vi "RefMem PtByPt Main Page.vi"(8 "error in (no error)":errorcluster, 11 "Node Ptr":T1 format="%.0x") -> (0 "error out":errorcluster)   [LabVIEW 2010, in "RefMem PtByPt Custom Device.lvlib"]
uses:
  RefMem PtByPt Custom Device.lvlib
  <vilib>/NI Veristand/Custom Device API/Custom Device Item Ref.ctl
  <vilib>/NI Veristand/Custom Device API/Path Specification.ctl
  <vilib>/NI Veristand/Custom Device API/Path Type.ctl
  <vilib>/NI Veristand/Custom Device API/Custom Device Execution Mode.ctl
  Controls/Data Channel Type.ctl
  <vilib>/NI Veristand/Custom Device API/Custom Device Channel.ctl
  <vilib>/NI Veristand/Custom Device API/Custom Device Channel Type.ctl
  Controls/Global.vi
  <vilib>/NI Veristand/Custom Device API/Get Item Property (String).vi
  <vilib>/NI Veristand/Custom Device API/Get Item Property (I32).vi
  <vilib>/NI Veristand/Custom Device API/Set Item Property (String).vi
  <vilib>/NI Veristand/Custom Device API/Set Item Property (U16).vi
  <vilib>/NI Veristand/Custom Device API/Set Item Property (I32).vi
  <vilib>/NI Veristand/Custom Device API/Custom Device API.lvlib
panel:
  in  "CPU Assignment":i32
  in  "Import":bool
  in  "Decimation":i32=1 min=1
  in  "VISA Name":string
  in  "Add Data Channel":bool
  in  "Add Data Folder":bool
  in  "Header":cluster{"Section Name":string}={"Section Name"="Reflective Memory Settings"}
  in  "Description":string
  in  "Name":string
  # "(-2 is Automatic)"
  # "(Only used if decimation >1)"
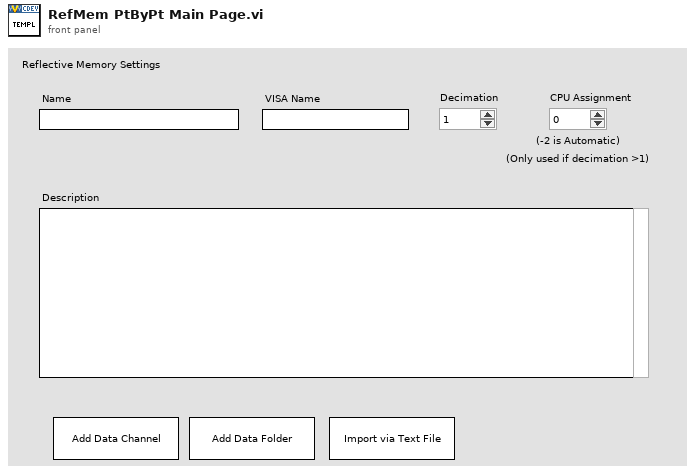
[diagram p1: front panel]
types:
  T1 = typedef "Custom Device API.lvlib/Custom Device Item Ref.ctl" = u64
  T2 = typedef "Custom Device API.lvlib/Custom Device Item Info.ctl" = cluster{"Name":string, "Is Channel":bool, "GUID":string}
  T3 = typedef "Custom Device API.lvlib/Path Specification.ctl" = cluster{"Path":path, "Type":T4}
  T4 = typedef "Custom Device API.lvlib/Path Type.ctl" = enum16{"Absolute", "To Base", "To Common Data Dir", "To Application Data Dir"}
  T5 = typedef "Custom Device API.lvlib/Custom Device Execution Mode.ctl" = enum16{"Asynchronous", "Inline HW Interface", "Inline Model Interface", "Inline Timing and Sync", "Asynchronous Timing and Sync"}
  T6 = typedef "RefMem PtByPt Custom Device.lvlib/Data Channel Type.ctl" = enum16{"Read", "Write"}
  T7 = typedef "Custom Device API.lvlib/Custom Device Channel.ctl" = cluster{"Type":T8, "Units":string, "Default Value":dbl, "Faultable":bool, "Scalable":bool}
  T8 = typedef "Custom Device API.lvlib/Custom Device Channel Type.ctl" = enum16{"Input", "Output"}
  T9 = typedef "Custom Device API.lvlib/Custom Device Commands.ctl" = enum16{"Default", "Item renamed", "Shutdown", "Dynamic button pressed"}
  T10 = typedef "Custom Device API.lvlib/Custom Device Pointer.ctl" = refnum<k24>
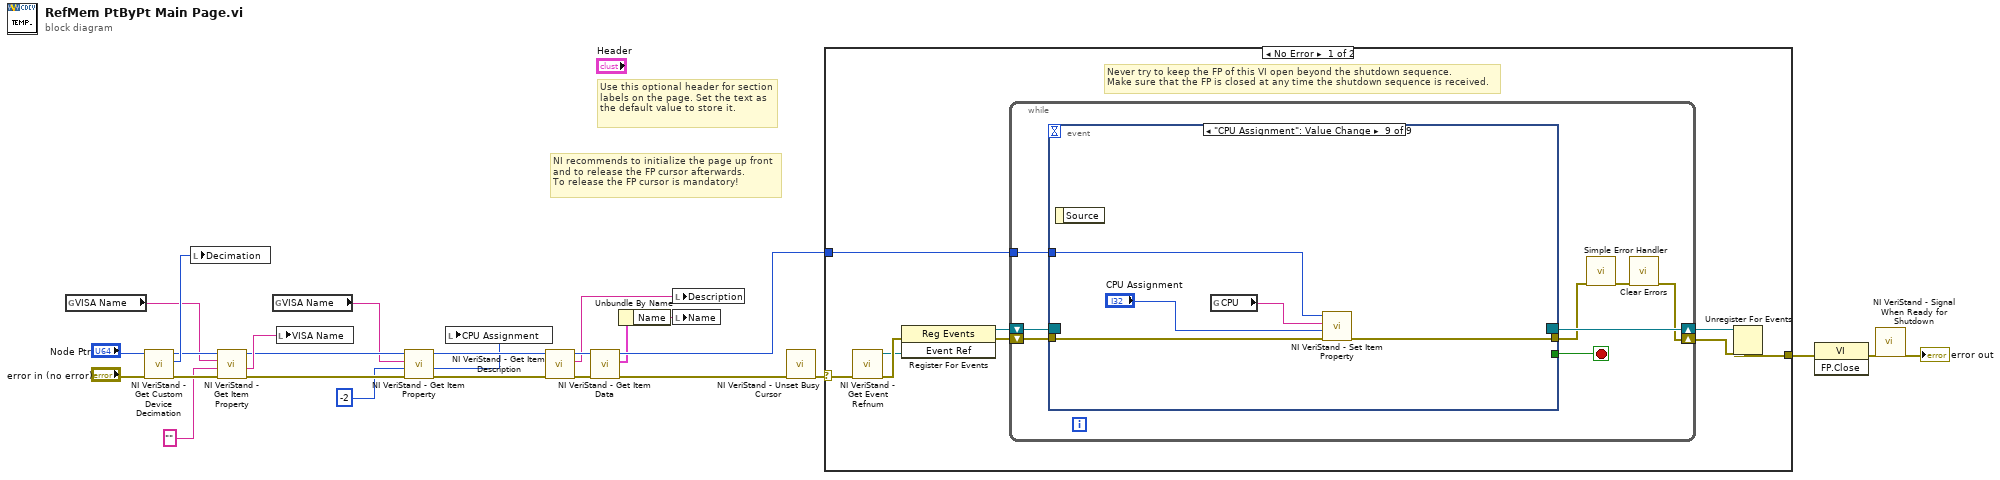
[diagram p0: block diagram]
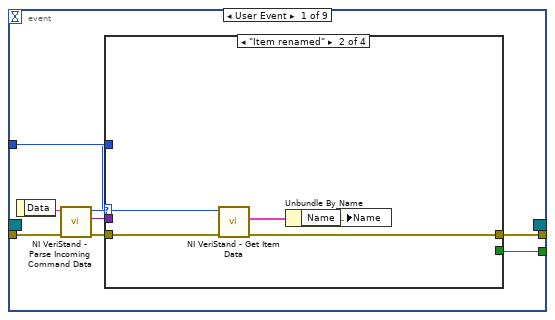
[diagram p2: hidden frame]
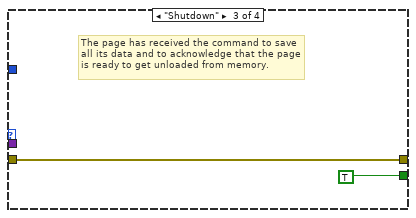
[diagram p4: hidden frame]
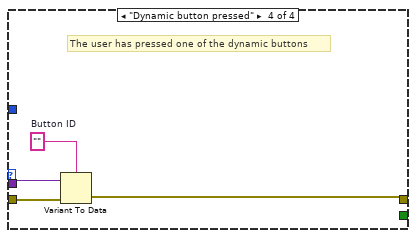
[diagram p5: hidden frame]
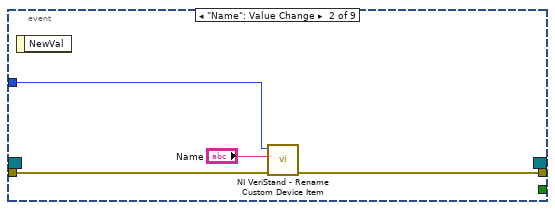
[diagram p6: hidden frame]
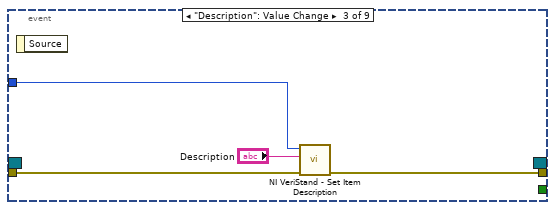
[diagram p7: hidden frame]
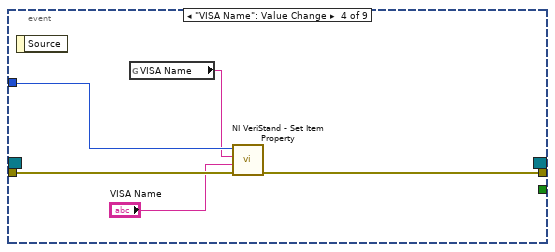
[diagram p8: hidden frame]
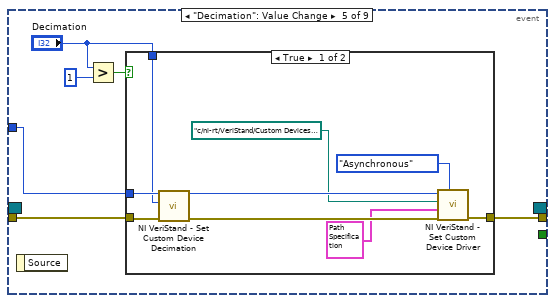
[diagram p9: hidden frame]
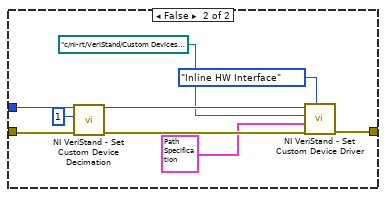
[diagram p10: hidden frame]
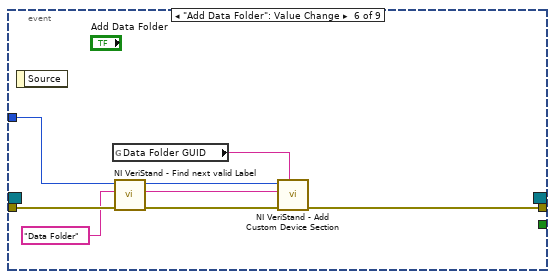
[diagram p11: hidden frame]
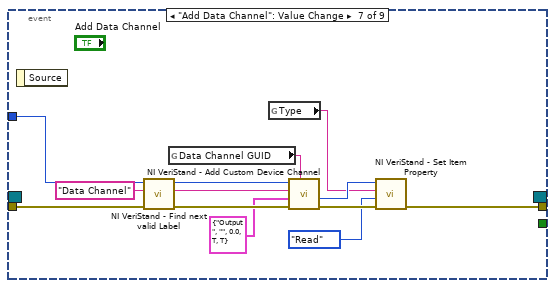
[diagram p12: hidden frame]
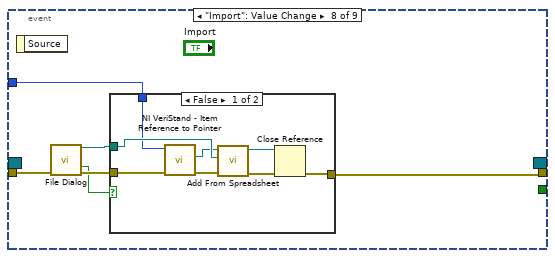
[diagram p13: hidden frame]
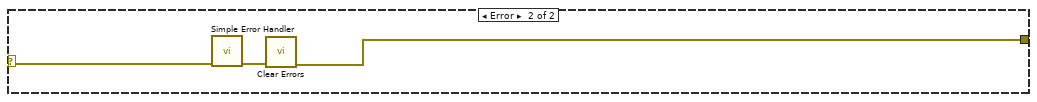
[diagram p15: hidden frame]
diagram:
  # "Use this optional header for section labels on the page. Set the text as the default value to store it."
  # "NI recommends to initialize the page up front\nand to release the FP cursor afterwards.\nTo release the FP cursor is mandatory!"
  n1 = global read "Global.vi" "VISA Name"() -> (w10:string)
  n2 = call <vilib>:"NI VeriStand - Get Custom Device Decimation.vi"("error in (no error)"="error in (no error)", "Device Ref in"="Node Ptr") -> ("error out"=w12:errorcluster, "Decimation"=w13:i32, "Device Ref out"=w11:T1)  [unwired: 7 in]
  n3 = local write "Decimation"(w13) -> ()
  n4 = call-poly <vilib>:"NI VeriStand - Get Item Property.vi"("error in (no error)"=w12, "Default Value"="" ("Section Name"), "Property Name"=w10, "Item Ref in"=w11) -> ("error out"=w7:errorcluster, "Value"=w8:string, "Item Ref out"=w6:T1)  [unwired: 4 in, 1 out]
  n5 = global read "Global.vi" "VISA Name"() -> (w5:string)
  n6 = local write "VISA Name"(w8) -> ()
  n7 = call-poly <vilib>:"NI VeriStand - Get Item Property.vi"("error in (no error)"=w7, "Default Value"=-2 ("CPU Assignment"), "Property Name"=w5, "Item Ref in"=w6) -> ("error out"=w3:errorcluster, "Value"=w1:i32, "Item Ref out"=w2:T1)  [unwired: 4 in, 1 out]
  n8 = local write "CPU Assignment"(w1) -> ()
  n9 = call <vilib>:"NI VeriStand - Get Item Description.vi"("error in (no error)"=w3, "Item Ref in"=w2) -> ("error out"=w18:errorcluster, "Description"=w19:string, "Item Ref out"=w20:T1)  [unwired: 7 out]
  n10 = call <vilib>:"NI VeriStand - Get Item Data.vi"("error in (no error)"=w18, "Item Ref in"=w20) -> ("error out"=w23:errorcluster, "Item Info"=w17:T2, "Item Ref out"=w21:T1)  [unwired: 7 out]
  n11 = Unbundle By Name(w17) -> ("Name"=w16:string)
  n12 = local write "Description"(w19) -> ()
  n13 = local write "Name"(w16) -> ()
  n14 = call <vilib>:"NI VeriStand - Unset Busy Cursor.vi"("error in (no error)"=w23) -> ("error out"=w22:errorcluster)  [unwired: 10 out]
  n15 = case shown="No Error" w22 {
    selector: w22 -> [w27 w144]
    tunnel: [w32 w142] -> w26
    tunnel: w21 -> [w28 _]
    frame No Error {
      # "Never try to keep the FP of this VI open beyond the shutdown sequence.\nMake sure that the FP is closed at any time the shutdown sequence is received."
      n16 = call <vilib>:"NI VeriStand - Get Event Refnum.vi"("error in (no error)"=w27) -> ("error out"=w35:errorcluster, "Event Ref"=w31:refnum<user-event>)  [unwired: 9 out]
      n17 = register-events(error in=w35, w31) -> (reference out=w29:refnum<event-registration>, error out=w30:errorcluster)  [unwired: 1 in]
      n18 = while {
        tunnel: w28 -> [w39]
        shift-right: [w36] -> w33
        shift-left: w30 -> [w42]
        shift-right: [w43] -> w34
        shift-left: w29 -> [w41]
        stop <- w40 stop-if-true
        n19 = event shown="[8] \"CPU Assignment\": Value Change" {
          selector: w41 -> [_ _ _ _ _ _ _ _ _]
          dyn-events: [_ _ _ _ _ _ _ _ _] -> w43
          timeout: _ -> [_ _ _ _ _ _ _ _ _]
          tunnel: w42 -> [w51 w67 w70 w76 w80 w106 w120 w127 w141]
          tunnel: [w47 _ _ _ _ _ _ _ _] -> w40
          tunnel: [w46 w66 w69 w74 w79 w107 w112 w124 w140] -> w38
          tunnel: w39 -> [w45 w65 w71 w75 w78 w105 w119 w122 w138]
          event User Event {
            n20 = event-data() -> ("Data"=w50:string)  [unwired: 1 out]
            n21 = call <vilib>:"NI VeriStand - Parse Incoming Command Data.vi"("error in (no error)"=w51, "Data"=w50) -> ("error out"=w49:errorcluster, "Data"=w44:variant, "Action"=w48:T9)  [unwired: 7 out]
            n22 = case shown="\"Item renamed\"" w48 {
              tunnel: w49 -> [w52 w57 w58 w63]
              tunnel: [_ _ TRUE _] -> w47
              tunnel: [w52 w54 w58 w60] -> w46
              tunnel: w45 -> [_ w56 _ _]
              tunnel: w44 -> [_ _ _ w62]
              frame "Default", Default {
              }
              frame "Item renamed" {
                n23 = call <vilib>:"NI VeriStand - Get Item Data.vi"("error in (no error)"=w57, "Item Ref in"=w56) -> ("error out"=w54:errorcluster, "Item Info"=w55:T2)  [unwired: 8 out]
                n24 = Unbundle By Name(w55) -> ("Name"=w53:string)
                n25 = local write "Name"(w53) -> ()
              }
              frame "Shutdown" {
                # "The page has received the command to save all its data and to acknowledge that the page is ready to get unloaded from memory."
              }
              frame "Dynamic button pressed" {
                w61 = ""  # Button ID
                # "The user has pressed one of the dynamic buttons"
                n26 = Variant To Data(error in=w63, Variant=w62, type=w61) -> (error out=w60:errorcluster)  [unwired: 1 out]
              }
            }
          }
          event "Name": Value Change {
            n27 = event-data() -> ()  [unwired: 2 out]
            n28 = call <vilib>:"NI VeriStand - Rename Custom Device Item.vi"("error in (no error)"=w67, "New Name"="Name", "Item Ref in"=w65) -> ("error out"=w66:errorcluster)  [unwired: 8 out]
          }
          event "Description": Value Change {
            n29 = event-data() -> ()  [unwired: 2 out]
            n30 = call <vilib>:"NI VeriStand - Set Item Description.vi"("error in (no error)"=w70, "Description"="Description", "Item Ref in"=w71) -> ("error out"=w69:errorcluster)  [unwired: 8 out]
          }
          event "VISA Name": Value Change {
            n31 = event-data() -> ()  [unwired: 2 out]
            n32 = global read "Global.vi" "VISA Name"() -> (w72:string)
            n33 = call-poly <vilib>:"NI VeriStand - Set Item Property.vi"("error in (no error)"=w76, "Value"="VISA Name", "Property Name"=w72, "Item Ref in"=w75) -> ("error out"=w74:errorcluster)  [unwired: 5 in, 2 out]
          }
          event "Decimation": Value Change {
            n34 = event-data() -> ()  [unwired: 2 out]
            n35 = Greater?(x="Decimation", y=u32 1) -> (0:w81:bool)
            n36 = case shown="True" w81 {
              tunnel: w80 -> [w89 w98]
              tunnel: [w91 w100] -> w79
              tunnel: w78 -> [w88 w97]
              tunnel: "Decimation" -> [w87 _]
              frame True {
                n37 = call <vilib>:"NI VeriStand - Set Custom Device Decimation.vi"("error in (no error)"=w89, "Decimation"=w87, "Device Ref in"=w88) -> ("error out"=w86:errorcluster, "Device Ref out"=w85:T1)  [unwired: 7 in]
                n38 = call <vilib>:"NI VeriStand - Set Custom Device Driver.vi"("Execution mode"=Custom_Device_Execution_Mode."Asynchronous", "error in (no error)"=w86, "Driver VI Path (Host)"=T3 {"Path"=path "Custom Devices/RefMem PtByPt/RefMem PtByPt Engine.llb/RefMem PtByPt RT Driver VI (Async).vi", "Type"=enum."To Common Data Dir"}, "Driver VI Path (RT)"=path "c:/ni-rt/VeriStand/Custom Devices/RefMem PtByPt/RefMem PtByPt Engine.llb/RefMem PtByPt RT Driver VI (Async).vi", "Device Ref in"=w85) -> ("error out"=w91:errorcluster)  [unwired: 5 in, 1 out]
              }
              frame False {
                n39 = call <vilib>:"NI VeriStand - Set Custom Device Decimation.vi"("error in (no error)"=w98, "Decimation"=1, "Device Ref in"=w97) -> ("error out"=w96:errorcluster, "Device Ref out"=w95:T1)  [unwired: 7 in]
                n40 = call <vilib>:"NI VeriStand - Set Custom Device Driver.vi"("Execution mode"=Custom_Device_Execution_Mode."Inline HW Interface", "error in (no error)"=w96, "Driver VI Path (Host)"=T3 {"Path"=path "Custom Devices/RefMem PtByPt/RefMem PtByPt Engine.llb/RefMem PtByPt RT Driver VI (Inline).vi", "Type"=enum."To Common Data Dir"}, "Driver VI Path (RT)"=path "c:/ni-rt/VeriStand/Custom Devices/RefMem PtByPt/RefMem PtByPt Engine.llb/RefMem PtByPt RT Driver VI (Inline).vi", "Device Ref in"=w95) -> ("error out"=w100:errorcluster)  [unwired: 5 in, 1 out]
              }
            }
          }
          event "Add Data Folder": Value Change {
            n41 = event-data() -> ()  [unwired: 2 out]
            n42 = global read "Global.vi" "Data Folder GUID"() -> (w108:string)
            n43 = call <vilib>:"NI VeriStand - Find next valid Label.vi"("error in (no error)"=w106, "Label"="Data Folder" ("Section Name"), "Item Ref in"=w105) -> ("error out"=w101:errorcluster, "Label out"=w102:string, "Item Ref out"=w104:T1)  [unwired: 4 in, 2 out]
            n44 = call <vilib>:"NI VeriStand - Add Custom Device Section.vi"("GUID (Default Section)"=w108, "error in (no error)"=w101, "Section Name"=w102, "Parent Ref in"=w104) -> ("error out"=w107:errorcluster)  [unwired: 4 in, 3 out]
          }
          event "Add Data Channel": Value Change {
            n45 = event-data() -> ()  [unwired: 2 out]
            n46 = call <vilib>:"NI VeriStand - Find next valid Label.vi"("error in (no error)"=w120, "Label"="Data Channel", "Item Ref in"=w119) -> ("error out"=w116:errorcluster, "Label out"=w118:string, "Item Ref out"=w117:T1)  [unwired: 4 in, 2 out]
            n47 = global read "Global.vi" "Data Channel GUID"() -> (w121:string)
            n48 = global read "Global.vi" "Type"() -> (w110:string)
            n49 = call <vilib>:"NI VeriStand - Add Custom Device Channel.vi"("GUID (Default Channel)"=w121, "error in (no error)"=w116, "Channel"=T7 {"Type"=enum."Output", "Units"="", "Default Value"=0.0, "Faultable"=TRUE, "Scalable"=TRUE}, "Channel Name"=w118, "Parent Ref in"=w117) -> ("error out"=w113:errorcluster, "Channel Ref"=w111:T1)  [unwired: 3 in, 2 out]
            n50 = call-poly <vilib>:"NI VeriStand - Set Item Property.vi"("error in (no error)"=w113, "Value"=Data_Channel_Type."Read" ("Type"), "Property Name"=w110, "Item Ref in"=w111) -> ("error out"=w112:errorcluster)  [unwired: 5 in, 2 out]
          }
          event "Import": Value Change {
            n51 = event-data() -> ()  [unwired: 2 out]
            n52 = call "File Dialog"("error in"=w127) -> ("selected path"=w125:path, "cancelled"=w123:bool, "error out"=w126:errorcluster)  [unwired: 11 in, 1 out]
            n53 = case shown="False" w123 {
              tunnel: w126 -> [w133 w136]
              tunnel: w122 -> [w134 _]
              tunnel: w125 -> [w135 _]
              tunnel: [w128 w136] -> w124
              frame False {
                n54 = call <vilib>:"NI VeriStand - Item Reference to Pointer.vi"("error in (no error)"=w133, "Item Ref in"=w134) -> ("error out"=w131:errorcluster, "Node Pointer"=w132:T10)  [unwired: 6 in, 2 out]
                n55 = call "Add From Spreadsheet.vi"("error in (no error)"=w131, "file path (use dialog)"=w135, "Device BaseNodeType in"=w132) -> ("error out"=w130:errorcluster, "Device BaseNodeType out"=w129:T10)  [unwired: 6 in, 1 out]
                n56 = Close Reference(reference=w129, error in (no error)=w130) -> (error out=w128:errorcluster)
              }
              frame True {
              }
            }
          }
          event "CPU Assignment": Value Change {
            n57 = event-data() -> ()  [unwired: 2 out]
            n58 = global read "Global.vi" "CPU"() -> (w139:string)
            n59 = call-poly <vilib>:"NI VeriStand - Set Item Property.vi"("error in (no error)"=w141, "Value"="CPU Assignment", "Property Name"=w139, "Item Ref in"=w138) -> ("error out"=w140:errorcluster)  [unwired: 5 in, 2 out]
          }
        }
        n60 = call <vilib>:"Simple Error Handler.vi"("error in (no error)"=w38) -> ("error out"=w37:errorcluster)  [unwired: 1 in, 7 out]
        n61 = call <vilib>:"Clear Errors.vi"("error in (no error)"=w37) -> ("error out"=w36:errorcluster)  [unwired: 6 out]
      }
      n62 = Unregister For Events(event registration refnum=w34, error in=w33) -> (error out=w32:errorcluster)
    }
    frame Error {
      n63 = call <vilib>:"Simple Error Handler.vi"("error in (no error)"=w144) -> ("error out"=w143:errorcluster)  [unwired: 1 in, 7 out]
      n64 = call <vilib>:"Clear Errors.vi"("error in (no error)"=w143) -> ("error out"=w142:errorcluster)  [unwired: 6 out]
    }
  }
  n65 = invoke class="VI" method="FP.Close"(error in=w26) -> (error out=w25:errorcluster)  [unwired: 2 in, 2 out]
  n66 = call <vilib>:"NI VeriStand - Signal When Ready for Shutdown.vi"("error in (no error)"=w25) -> ("error out"=→"error out":errorcluster)  [unwired: 10 out]
